vi "Init.vi"(6 "Number of devices":i32=1, 8 "error in (no error)":errorcluster, 9 "Head Device No":string="000", 10 "Device Type":string="D", 11 "Device in":refnum<class "Device.lvclass">) -> (0 "error out":errorcluster, 3 "Device out":refnum<class "Device.lvclass">)   [LabVIEW 2019, in "SLMP.lvlib" / "Device.lvclass"]
uses:
  Device.lvclass
  Device.lvclass/Device.ctl
  601cd0db-5801-40fa-bebb-2b4fbe7ef0d3.vi
  2fe85cd6-8f41-4664-8daa-7f3f22a3bb8b.vi
  <vilib>/JDP Science/JSONtext/Variant to JSON Text.vi
  <vilib>/JDP Science/JSONtext/LVClass Serializer/JSONtext LVClass Serializer.lvclass
  <vilib>/JDP Science/JSONtext/JSONtext.lvlib
panel:
  out "Device":string
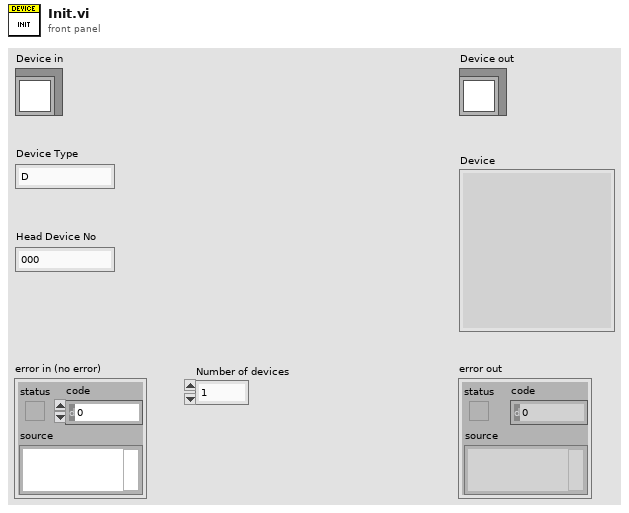
[diagram p1: front panel]
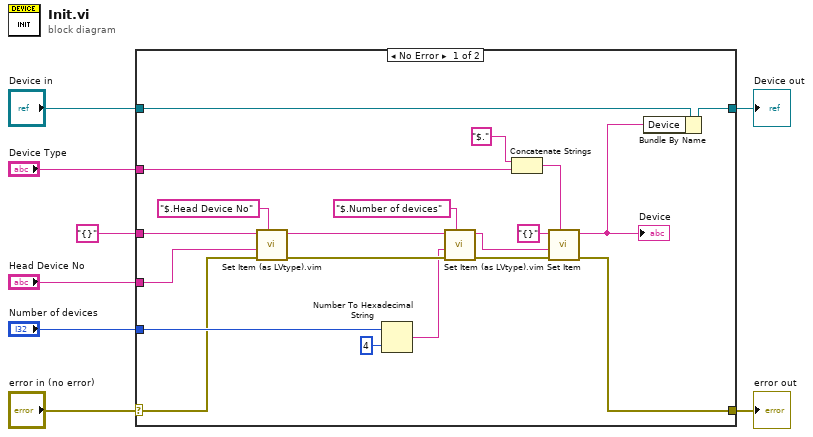
[diagram p0: block diagram]
diagram:
  n1 = case shown="No Error" "error in (no error)" {
    selector: "error in (no error)" -> [w10 w30]
    tunnel: [w9 w30] -> w7
    tunnel: [w12 w29] -> w5
    tunnel: "Device in" -> [w28 w29]
    tunnel: "Head Device No" -> [w27 _]
    tunnel: "Number of devices" -> [w22 _]
    tunnel: "{}" -> [w19 _]
    tunnel: "Device Type" -> [w15 _]
    frame No Error {
      n2 = call "Set Item (as LVtype).vim"("Object (or Item) Path"="$.Head Device No" ("$Path or Item Name"), "error in (no error)"=w10, "Anything"=w27, "JSON"=w19) -> ("error out"=w25:errorcluster, "<JSON>"=w24:string)  [unwired: 4 in, 1 out]
      n3 = Number To Hexadecimal String(1:i16 4 ("width (-)"), 2:w22) -> (0:w20:string)
      n4 = call "Set Item (as LVtype).vim"("Object (or Item) Path"="$.Number of devices", "error in (no error)"=w25, "Anything"=w20, "JSON"=w24) -> ("error out"=w18:errorcluster, "<JSON>"=w17:string)  [unwired: 4 in, 1 out]
      n5 = Concatenate Strings("$." ("$Path or Item Name"), w15) -> (w13:string)
      n6 = call <vilib>:"Set Item.vi"("$Path or Item Name"=w13, "error in (no error)"=w18, "JSON to Insert"=w17, "JSON"="{}") -> ("error out"=w9:errorcluster, "<JSON>"=w11:string)  [unwired: 4 in, 1 out]
      "Device" <- w11
      n7 = Bundle By Name(cluster=w28, "Device"=w11) -> (w12:refnum<class "Device.lvclass">)
    }
    frame Error {
    }
  }
  "error out" <- w7
  "Device out" <- w5
